vi "On Change Configuation Path.vi"(8 "error in (no error)":errorcluster, 10 "Path":path, 11 "App in":refnum<class "App.lvclass">) -> (0 "error out":errorcluster, 3 "App out":refnum<class "App.lvclass">)   [LabVIEW 2020, in "AR Example.lvlib" / "App.lvclass"]
uses:
  App.lvclass
  g_ar_toolkit.common/Camera Matrix.ctl
  g_ar_toolkit.common/Camera Distortion Coefficients.ctl
  g_ar_toolkit.common/Camera Parameters.ctl
  JSON Configuration Data.ctl
  UI/UI.lvclass
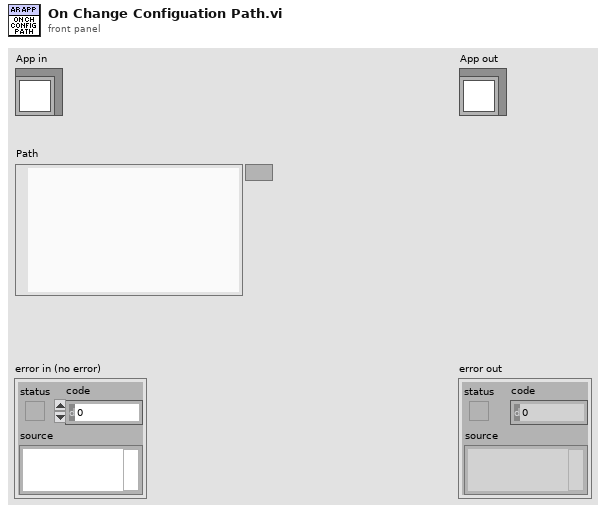
[diagram p1: front panel]
types:
  T1 = typedef "AR Example.lvlib/App.lvclass/JSON Configuration Data.ctl" = cluster{"Version":u32, "Camera Name":string, "Camera Parameters":T2, "Reprojection Error":dbl, "Timestamp":string}
  T2 = typedef "g_ar_toolkit.common.lvlib/Camera Parameters.ctl" = cluster{"Matrix":T3, "Distortion":T4}
  T3 = typedef "g_ar_toolkit.common.lvlib/Camera Matrix.ctl" = cluster{"m 0,0":dbl, "m 0,1":dbl, "m 0,2":dbl, "m 1,0":dbl, "m 1,1":dbl, "m 1,2":dbl, "m 2,0":dbl, "m 2,1":dbl, "m 2,2":dbl}
  T4 = typedef "g_ar_toolkit.common.lvlib/Camera Distortion Coefficients.ctl" = cluster{"k1":dbl, "k2":dbl, "p1":dbl, "p2":dbl, "k3":dbl, "k4":dbl, "k5":dbl, "k6":dbl, "s1":dbl, "s2":dbl, "s3":dbl, "s4":dbl, "tau x":dbl, "tau y":dbl}
  T5 = typedef "AR Example.lvlib/App.lvclass/JSON Configuration Data.ctl" = cluster{"Version":u32, "Camera Name":string, "Camera Parameters":T2, "Reprojection Error":dbl, "Timestamp":string, "Image Size":T6}
  T6 = typedef "g_ar_toolkit.common.lvlib/Image Size (Integer).ctl" = cluster{"Width":u16, "Height":u16}
  T7 = cluster{"Configuration Data":T1, "appended path":path}
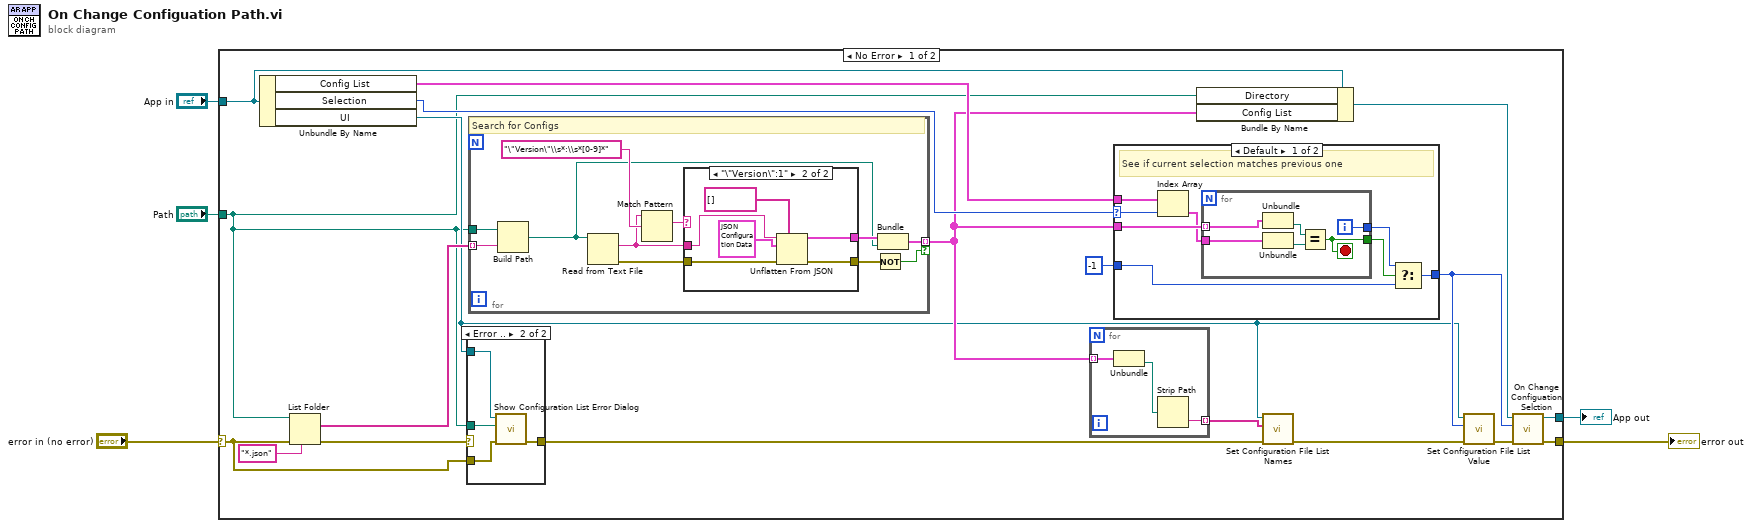
[diagram p0: block diagram]
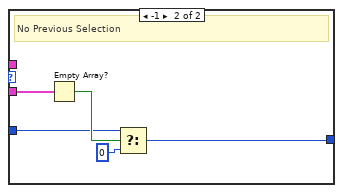
[diagram p3: hidden frame]
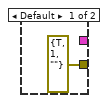
[diagram p4: hidden frame]
diagram:
  n1 = case shown="No Error" "error in (no error)" {
    selector: "error in (no error)" -> [w10 w70]
    tunnel: [w18 w71] -> w4
    tunnel: "Path" -> [w8 _]
    tunnel: [w17 w70] -> w2
    tunnel: "App in" -> [w16 w71]
    frame No Error {
      n2 = Unbundle By Name(w16) -> ("Config List"=w21:cluster{"Data":T5, "Source":path}[], "Selection"=w22:i32, "UI"=w9:refnum<class "UI.lvclass">)
      n3 = List Folder(path=w8, pattern="*.json", error in=w10) -> (filenames=w23:string[], error out=w7:errorcluster)  [unwired: 1 in, 2 out]
      n4 = case shown="Error .." w7 {
        selector: w7 -> [w25 _]
        tunnel: w10 -> [_ w29]
        tunnel: w9 -> [_ w28]
        tunnel: w8 -> [_ w27]
        tunnel: [w25 w26] -> w6
        frame No Error {
        }
        frame Error {
          n5 = call-dynamic "Show Configuration List Error Dialog.vi"("error in (no error)"=w29, "Value"=w27, "UI in"=w28) -> ("error out"=w26:errorcluster)  [unwired: 8 in]
        }
      }
      n6 = for {
        tunnel: w23 -> [w54] mode=indexing
        tunnel: [w56] -> w15 mode=indexing if=w57
        tunnel: w8 -> [w55]
        # "Search for Configs"
        n7 = Build Path(base path=w55, name or relative path=w54) -> (appended path=w52:path)
        n8 = Read from Text File(file (use dialog)=w52) -> (text=w58:string, error out=w59:errorcluster)  [unwired: 3 in, 2 out]
        n9 = Match Pattern(string=w58, regular expression="\"Version\"\\s*:\\s*[0-9]*") -> (match substring=w61:string)  [unwired: 1 in, 3 out]
        n10 = case shown="\"\\\"Version\\\":1\"" w61 {
          tunnel: w59 -> [_ w69]
          tunnel: [_ w68] -> w53
          tunnel: [errorcluster {"status"=TRUE, "code"=1, "source"=""} ("error out") w67] -> w60
          tunnel: w58 -> [_ w65]
          frame Default {
          }
          frame "\"Version\":1" {
            n11 = Unflatten From JSON(path=string[] [], JSON string=w65, type and defaults=T1 {"Version"=0, "Camera Name"="", "Camera Parameters"={"Matrix"={"m 0,0"=0.0, "m 0,1"=0.0, "m 0,2"=0.0, "m 1,0"=0.0, "m 1,1"=0.0, "m 1,2"=0.0, "m 2,0"=0.0, "m 2,1"=0.0, "m 2,2"=0.0}, "Distortion"={"k1"=0.0, "k2"=0.0, "p1"=0.0, "p2"=0.0, "k3"=0.0, "k4"=0.0, "k5"=0.0, "k6"=0.0, "s1"=0.0, "s2"=0.0, "s3"=0.0, "s4"=0.0, "tau x"=0.0, "tau y"=0.0}}, "Reprojection Error"=0.0, "Timestamp"=""} ("Configuration Data"), error in (no error)=w69) -> (value=w68:T1, error out=w67:errorcluster)  [unwired: 3 in]
          }
        }
        n12 = Not(x=w60) -> (.not. x?=w57:bool)
        n13 = Bundle("Configuration Data"=w53, "appended path"=w52) -> (w56:T7)  [unwired: 1 in]
      }
      n14 = for {
        tunnel: w15 -> [w32] mode=indexing
        tunnel: [w30] -> w14 mode=indexing
        n15 = Unbundle(w32) -> ("appended path"=w31:path)  [unwired: 1 out]
        n16 = Strip Path(path=w31) -> (name=w30:string)  [unwired: 1 out]
      }
      n17 = case shown="Default" w22 {
        selector: w22 -> [w39 _]
        tunnel: w21 -> [w40 _]
        tunnel: w15 -> [w38 w51]
        tunnel: -1 ("f") -> [w34 w49]
        tunnel: [w33 w47] -> w11
        frame Default {
          # "See if current selection matches previous one"
          n18 = Index Array(array=w40, index=w39) -> (element=w37:cluster{"Data":T5, "Source":path})
          n19 = for {
            tunnel: w38 -> [w44] mode=indexing
            tunnel: w37 -> [w45]
            tunnel: [w46] -> w36
            tunnel: [w41] -> w35
            i -> [w46]
            stop <- w41 stop-if-true
            n20 = Unbundle(w44) -> ("appended path"=w43:path)  [unwired: 1 out]
            n21 = Unbundle(w45) -> ("Source"=w42:path)  [unwired: 1 out]
            n22 = Equal?(x=w43, y=w42) -> (x = y?=w41:bool)
          }
          n23 = Select(t=w36, s=w35, f=w34) -> (s? t:f=w33:i32)
        }
        frame -1 {
          # "No Previous Selection"
          n24 = Empty Array?(array=w51) -> (empty?=w50:bool)
          n25 = Select(t=w49, s=w50, f=0) -> (s? t:f=w47:i32)
        }
      }
      n26 = Bundle By Name(cluster=w16, "Directory"=w8, "Config List"=w15) -> (w19:refnum<class "App.lvclass">)
      n27 = call-dynamic "Set Configuration File List Names.vi"("error in (no error)"=w6, "Values"=w14, "UI in"=w9) -> ("error out"=w13:errorcluster)  [unwired: 8 in]
      n28 = call-dynamic "Set Configuration File List Value.vi"("error in (no error)"=w13, "Value"=w11, "UI in"=w9) -> ("error out"=w12:errorcluster)  [unwired: 8 in]
      n29 = call "On Change Configuation Selction.vi"("error in (no error)"=w12, "Selection"=w11, "App in"=w19) -> ("error out"=w17:errorcluster, "App out"=w18:refnum<class "App.lvclass">)  [unwired: 7 in]
    }
    frame Error {
    }
  }
  "App out" <- w4
  "error out" <- w2
